vi "unbuffered_waveform_graph.vi"() -> ()   [LabVIEW 2019]
panel:
  in  "stop":bool
  out "Waveform Graph":i32[](graph)
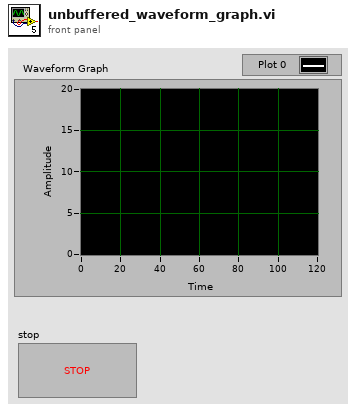
[diagram p1: front panel]
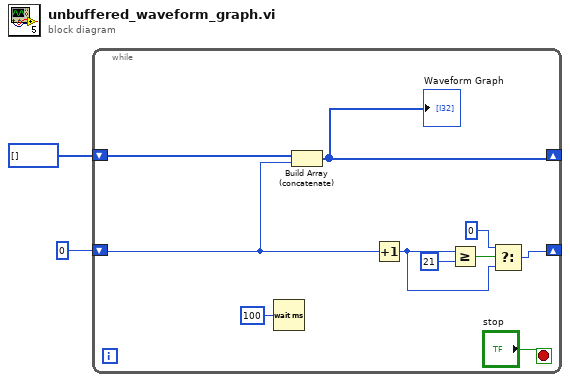
[diagram p0: block diagram]
diagram:
  n1 = while {
    shift-right: [w8] -> _
    shift-left: 0 -> [w5]
    shift-right: [w4] -> _
    shift-left: i32[] [] -> [w6]
    stop <- "stop" stop-if-true
    n2 = Wait (ms)(milliseconds to wait=u32 100) -> ()  [unwired: 1 out]
    n3 = Build Array (concatenate)(w6, w5) -> (w4:i32[])
    "Waveform Graph" <- w4
    n4 = Increment(x=w5) -> (x+1=w9:i32)
    n5 = Greater Or Equal?(x=w9, y=21) -> (x >= y?=w11:bool)
    n6 = Select(t=0 ("y"), s=w11, f=w9) -> (s? t:f=w8:i32)
  }
